vi "SuperSampleMaster2.vi"() -> ()   [LabVIEW 2012]
doc: "A sample master that can be run on the computer or RIO"
uses:
  <userlib>/ROS for LabVIEW Software/ROS/Code/SubVIs/_ROSDirection.ctl
  <userlib>/ROS for LabVIEW Software/ROS/Code/Console/Servers/ServerSubs/TopicDef.ctl
  <userlib>/ROS for LabVIEW Software/ROS/MessageBuilding/std_msgs/subs/stringScalar.vi
  <userlib>/ROS for LabVIEW Software/ROS/MessageParsing/std_msgs/subs/parse_string_scalar.vi
panel:
  in  "Service call":bool
  out "Reply":string
  out "time":string
  out "Status":string
  in  "stop":bool
  # "Instructions:\n1. Run the VI\n2. Verify that you see the correct time.\n3. Press the LED button. You should see the LED reply change.\nIf you are targetting a myRIO, the LED should change as well.\n4. Debug by clicking Show Node and Show Webpage.\n5. See what is being sent back and forth by clicking Show Node and Show Webpage."
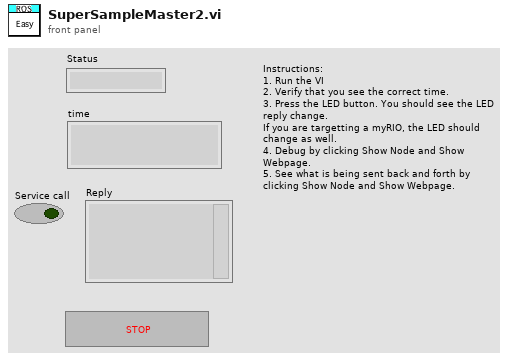
[diagram p1: front panel]
types:
  T1 = typedef "TopicDef.ctl" = cluster{"Topic":string, "Type":string, "Action":T2, "Update (ms)":u16, "queue size":u16}
  T2 = typedef "_ROSDirection.ctl" = enum16{"Node", "Publisher", "Subscriber", "ServiceClient", "ServiceProvider"}
  T3 = cluster{"Topic":string, "Type":string, "Action":T2, "Update (ms)":u16, "queue":u16}
  T4 = typedef "_ROSControl.ctl" = cluster{"topic port":u16, "Node":string, "topic":string, "type":string, "node port":u16, "error ":errorcluster, "Direction":T2, "Update (ms)":u16, "FIFO size":u16}
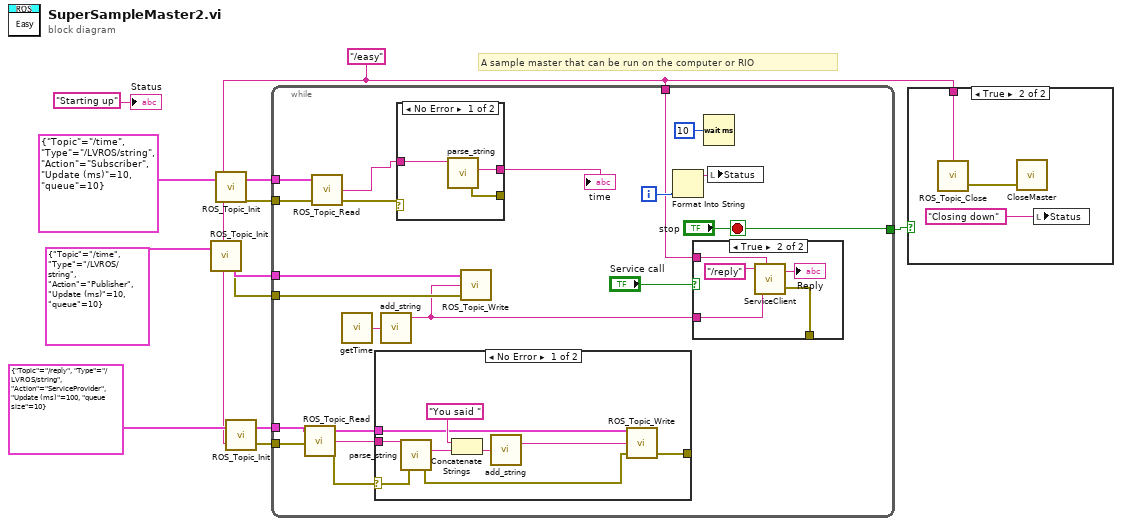
[diagram p0: block diagram]
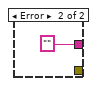
[diagram p5: hidden frame]
diagram:
  w1 = "/easy" ("Topic")
  # "A sample master that can be run on the computer or RIO"
  n1 = call <userlib>:"ROS_Topic_Init.vi"("node"=w1, "Definitions"=T3 {"Topic"="/time", "Type"="/LVROS/string", "Action"=enum."Publisher", "Update (ms)"=10, "queue"=10}) -> ("error out"=w6:errorcluster, "ROS out"=w7:T4)
  n2 = call <userlib>:"ROS_Topic_Init.vi"("node"=w1, "Definitions"=T3 {"Topic"="/time", "Type"="/LVROS/string", "Action"=enum."Subscriber", "Update (ms)"=10, "queue"=10}) -> ("error out"=w5:errorcluster, "ROS out"=w9:T4)
  n3 = call <userlib>:"ROS_Topic_Init.vi"("node"=w1, "Definitions"=T1 {"Topic"="/reply", "Type"="/LVROS/string", "Action"=enum."ServiceProvider", "Update (ms)"=100, "queue size"=10}) -> ("error out"=w2:errorcluster, "ROS out"=w3:T4)
  n4 = while {
    tunnel: ["stop"] -> w11
    tunnel: w9 -> [w28]
    tunnel: w7 -> [w24]
    tunnel: w6 -> [w23]
    tunnel: w5 -> [w22]
    tunnel: w3 -> [w18]
    tunnel: w2 -> [w17]
    tunnel: w1 -> [w14]
    i -> [w29]
    stop <- "stop" stop-if-true
    n5 = call <userlib>:"ROS_Topic_Read.vi"("error in (no error)"=w17, "ROS in"=w18) -> ("error out"=w16:errorcluster, "Reply"=w19:string, "ROS out"=w20:T4)  [unwired: 1 in]
    n6 = call <userlib>:"ROS_Topic_Read.vi"("error in (no error)"=w22, "ROS in"=w28) -> ("error out"=w26:errorcluster, "Reply"=w27:string)  [unwired: 1 in, 1 out]
    n7 = call <userlib>:"getTime.vi"() -> ("Current Time"=w21:string)  [unwired: 1 in]
    n8 = case shown="No Error" w16 {
      selector: w16 -> [w39 _]
      tunnel: w20 -> [w43 _]
      tunnel: w19 -> [w42 _]
      tunnel: [w41 _] -> _
      frame No Error {
        n9 = call-poly <userlib>:"parse_string.vi"("error in"=w39, "msg in"=w42) -> ("error out"=w38:errorcluster, "string"=w44:string)  [unwired: 3 in, 1 out]
        n10 = Concatenate Strings("You said " ("string"), w44) -> (w45:string)
        n11 = call-poly <userlib>:"add_string.vi"("String"=w45) -> ("msg out"=w40:string)  [unwired: 4 in]
        n12 = call <userlib>:"ROS_Topic_Write.vi"("error in (no error)"=w38, "Msg in"=w40, "ROS in"=w43) -> ("error out"=w41:errorcluster)  [unwired: 1 in, 1 out]
      }
      frame Error {
      }
    }
    n13 = call-poly <userlib>:"add_string.vi"("String"=w21) -> ("msg out"=w15:string)  [unwired: 4 in]
    n14 = case shown="No Error" w26 {
      tunnel: w27 -> [w49 _]
      tunnel: [w48 "" ("string")] -> w25
      tunnel: [w47 _] -> _
      frame No Error {
        n15 = call-poly <userlib>:"parse_string.vi"("msg in"=w49) -> ("error out"=w47:errorcluster, "string"=w48:string)  [unwired: 4 in, 1 out]
      }
      frame Error {
      }
    }
    "time" <- w25
    n16 = call <userlib>:"ROS_Topic_Write.vi"("error in (no error)"=w23, "Msg in"=w15, "ROS in"=w24) -> ()  [unwired: 1 in, 2 out]
    n17 = Format Into String(w29) -> (resulting string=w31:string)  [unwired: 3 in, 1 out]
    n18 = case shown="True" "Service call" {
      tunnel: w15 -> [_ w37]
      tunnel: w14 -> [_ w36]
      tunnel: [_ w34] -> _
      frame False {
      }
      frame True {
        n19 = call <userlib>:"ServiceClient.vi"("Topic"="/reply", "node"=w36, "Msg in"=w37) -> ("Reply"=→"Reply":string, "error out"=w34:errorcluster)  [unwired: 2 in]
      }
    }
    n20 = Wait (ms)(milliseconds to wait=u32 10) -> ()  [unwired: 1 out]
    n21 = local write "Status"(w31) -> ()
  }
  n22 = case shown="True" w11 {
    tunnel: w1 -> [_ w52]
    frame False {
    }
    frame True {
      n23 = call <userlib>:"ROS_Topic_Close.vi"("node"=w52) -> ("error out"=w51:errorcluster)  [unwired: 3 in]
      n24 = call <userlib>:"CloseMaster.vi"("error in (no error)"=w51) -> ()  [unwired: 2 in, 1 out]
      n25 = local write "Status"("Closing down" ("Status")) -> ()
    }
  }
  "Status" <- "Starting up" ("Status")
